vi "Update Entity OoC.vi"(7 "Type Path Map":map{path, path}(c390), 8 "error in (no error)":errorcluster, 9 "Definition":T1[](array[typedef]), 10 "Entity Path":path, 11 "Project Ref":refnum<vi>) -> (0 "error out":errorcluster)   [LabVIEW 2020, in "Conditum-Tools.lvlib" / "Entity Editor.lvclass"]
uses:
  Entity Editor.lvclass
  Field Config.ctl
  Conditum-Clone/Columns/Type/Type.lvclass
  Accessors.ctl
  Accessor Scope.ctl
  Conditum-Clone/Columns/Type/Type.lvclass/Type.ctl
  Conditum-Tools.lvlib
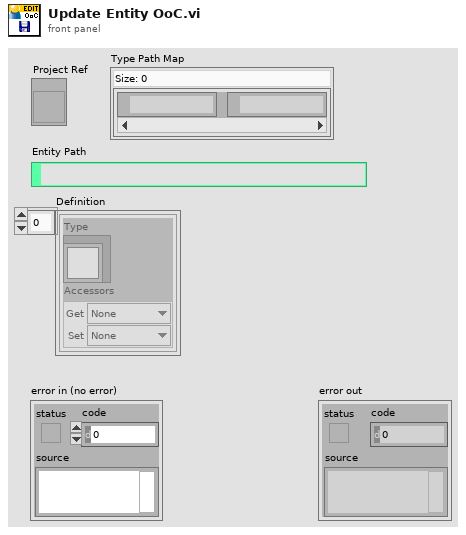
[diagram p1: front panel]
types:
  T1 = typedef "Conditum-Tools.lvlib/Field Config.ctl" = cluster{"Type":refnum<class "Type.lvclass">, "Accessors":T2}
  T2 = typedef "Conditum-Tools.lvlib/Accessors.ctl" = cluster{"Get":T3, "Set":T3}
  T3 = typedef "Conditum-Tools.lvlib/Accessor Scope.ctl" = enum16{"None", "Public", "Protected", "Private"}
  T4 = typedef "Conditum-Tools.lvlib/Entity Editor.lvclass/Entity Paths.ctl" = cluster{"LVClass":path, "Columns.ctl":path, "Columns.vi":path, "Set Defaults.vi":path, "Update All Values.vi":path}
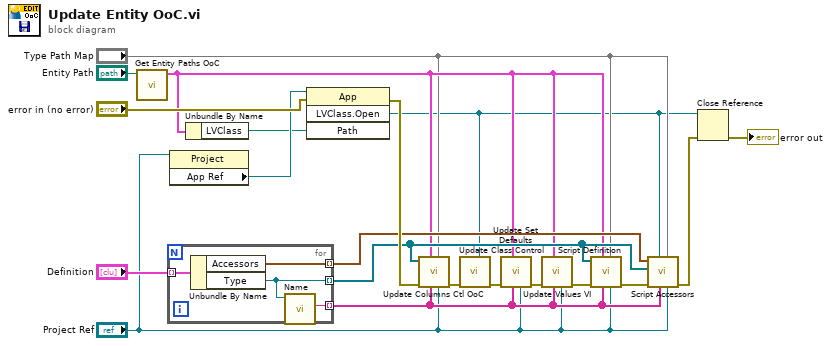
[diagram p0: block diagram]
diagram:
  n1 = call "Get Entity Paths OoC.vi"("Entity Path"="Entity Path") -> ("Entity Paths"=w6:T4)  [unwired: 10 in]
  n2 = for {
    tunnel: "Definition" -> [w24] mode=indexing
    tunnel: [w23] -> w4 mode=indexing
    tunnel: [w22] -> w8 mode=indexing
    tunnel: [w21] -> w7 mode=indexing
    n3 = Unbundle By Name(w24) -> ("Accessors"=w21:T2, "Type"=w22:refnum<class "Type.lvclass">)
    n4 = call "Name.vi"("Type in"=w22) -> ("Table Name"=w23:string)  [unwired: 10 in]
  }
  n5 = property class="Project"(reference="Project Ref") -> ("App Ref"=w15:refnum<vi>)  [unwired: 1 in, 2 out]
  n6 = Unbundle By Name(w6) -> ("LVClass"=w14:path)
  n7 = invoke class="App" method="LVClass.Open"(reference=w15, error in="error in (no error)", "Path"=w14) -> (error out=w20:errorcluster, "LVClass.Open"=w1:refnum<vi>)  [unwired: 1 in, 2 out]
  n8 = call "Update Columns Ctl OoC.vi"("Project Ref"="Project Ref", "Type Path Map"="Type Path Map", "Names"=w4, "Entity Paths"=w6, "error in (no error)"=w20, "Updated Definition"=w8) -> ("error"=w17:errorcluster)  [unwired: 5 in]
  n9 = call "Update Class Control.vi"("LVClass"=w1, "error in (no error)"=w17) -> ("error out"=w16:errorcluster)  [unwired: 9 in]
  n10 = call "Update Set Defaults.vi"("Project Ref"="Project Ref", "Names"=w4, "Entity Paths"=w6, "error in (no error)"=w16) -> ("error"=w12:errorcluster)  [unwired: 7 in]
  n11 = call "Update Values VI.vi"("Project Ref"="Project Ref", "Names"=w4, "Entity Paths"=w6, "error in (no error)"=w12) -> ("error"=w11:errorcluster)  [unwired: 7 in]
  n12 = call "Script Definition.vi"("Project Ref"="Project Ref", "Type Path Map"="Type Path Map", "Names"=w4, "Entity Paths"=w6, "error in (no error)"=w11, "Updated Definition"=w8) -> ("error"=w9:errorcluster)  [unwired: 5 in]
  n13 = call "Script Accessors.vi"("Project Ref"="Project Ref", "Type Path Map"="Type Path Map", "Names"=w4, "LVClass"=w1, "error in (no error)"=w9, "Updated Definition"=w8, "Accessors"=w7) -> ("error"=w2:errorcluster)  [unwired: 4 in]
  n14 = Close Reference(reference=w1, error in (no error)=w2) -> (error out=→"error out":errorcluster)
